vi "User32dllAPI.MaxWindow.vi"(8 "error in (no error)":errorcluster, 11 "hWnd":i32) -> (0 "error out":errorcluster, 3 "hWnd out":i32)   [LabVIEW 2015]
uses:
  user32.dll
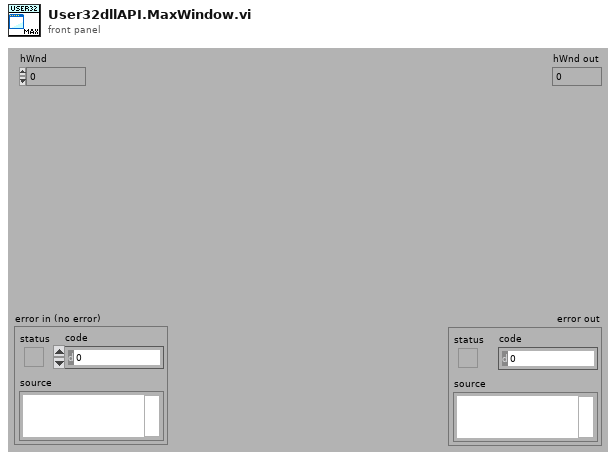
[diagram p1: front panel]
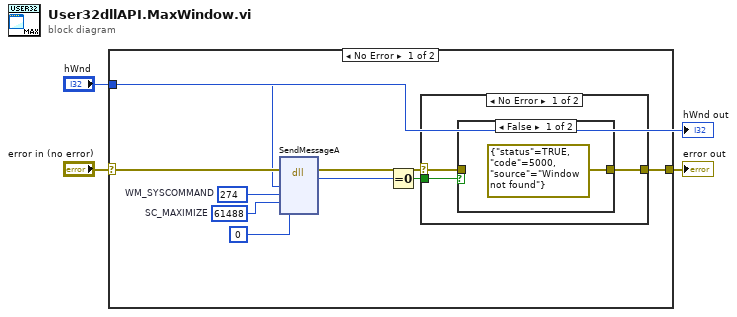
[diagram p0: block diagram]
diagram:
  n1 = case shown="No Error" "error in (no error)" {
    selector: "error in (no error)" -> [w9 w19]
    tunnel: [w11 w19] -> w2
    tunnel: "hWnd" -> [w6 _]
    frame No Error {
      w5 = 61488  # SC_MAXIMIZE
      w10 = u32 274  # WM_SYSCOMMAND
      n2 = dll-call lib="USER32.DLL" fn="SendMessageA" label="SendNotifyMessage"(error in=w9, "hWnd"=w6, "Msg"=w10, "wParam"=w5, "lParam"=0) -> (error out=w8:errorcluster, "result"=w7:i32)  [unwired: 6 in, 1 out]
      n3 = Equal To 0?(x=w7) -> (x = 0?=w12:bool)
      n4 = case shown="No Error" w8 {
        selector: w8 -> [w13 w18]
        tunnel: w12 -> [w15 _]
        tunnel: [w14 w18] -> w11
        frame No Error {
          n5 = case shown="False" w15 {
            tunnel: [errorcluster {"status"=TRUE, "code"=5000, "source"="Window not found"} ("error out") w17] -> w14
            tunnel: w13 -> [_ w17]
            frame False {
            }
            frame True {
            }
          }
        }
        frame Error {
        }
      }
    }
    frame Error {
    }
  }
  "error out" <- w2
  "hWnd out" <- "hWnd"
